vi "m1m3_monitorCommand_ApplyAOSCorrectionByForces.vi"(8 "error in (no error)":errorcluster, 11 "command_ApplyAOSCorrectionByForces_Ctl":T1) -> (0 "error out":errorcluster, 2 "function return":i32, 3 "command_ApplyAOSCorrectionByForces_Ctl out":T1)   [LabVIEW 2016, in "SALLV_m1m3.lvlib"]
doc: "int m1m3_shm_monitorCommand_ApplyAOSCorrectionByForcesLV(m1m3_command_ApplyAOSCorrectionByForcesLV *command_ApplyAOSCorrectionByForces_Ctl );"
uses:
  SALLV_m1m3.lvlib
  DataTypes/command_ApplyAOSCorrectionByForces.ctl
  SALLV_m1m3.so
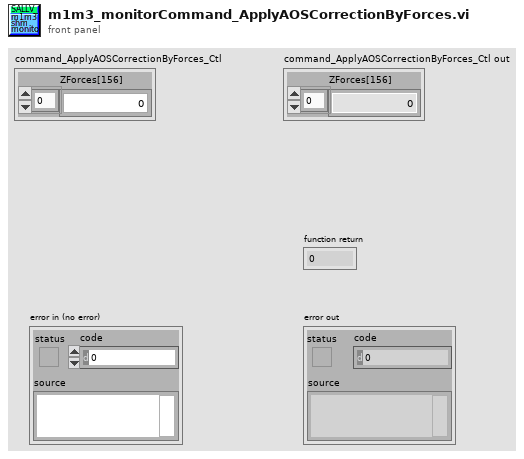
[diagram p1: front panel]
types:
  T1 = typedef "SALLV_m1m3.lvlib/command_ApplyAOSCorrectionByForces.ctl" = cluster{"ZForces[156]":dbl[]}
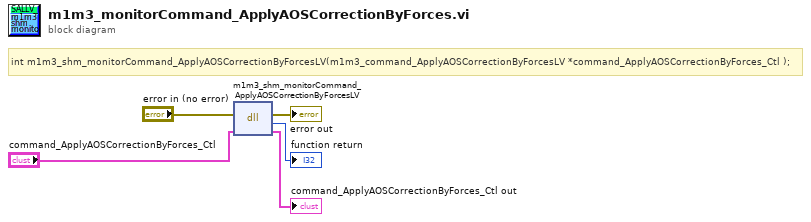
[diagram p0: block diagram]
diagram:
  # "int m1m3_shm_monitorCommand_ApplyAOSCorrectionByForcesLV(m1m3_command_ApplyAOSCorrectionByForcesLV *command_ApplyAOSCorrectionByForces_Ctl );"
  n1 = dll-call lib="opt/CODE/SALLV_m1m3/SALLV_m1m3.*" fn="m1m3_shm_monitorCommand_ApplyAOSCorrectionByForcesLV"(error in="error in (no error)", "command_ApplyAOSCorrectionByForces_Ctl"="command_ApplyAOSCorrectionByForces_Ctl") -> (error out=→"error out":errorcluster, →"function return":i32, "command_ApplyAOSCorrectionByForces_Ctl"=→"command_ApplyAOSCorrectionByForces_Ctl out":T1)  [unwired: 2 in, 1 out]
